vi "数组波形.vi"() -> ()   [LabVIEW 2018]
uses:
  <vilib>/measure/NI_MABase.lvlib
panel:
  out "Dynamic Data Type":dynamicdata(graph) caption="动态数据类型"
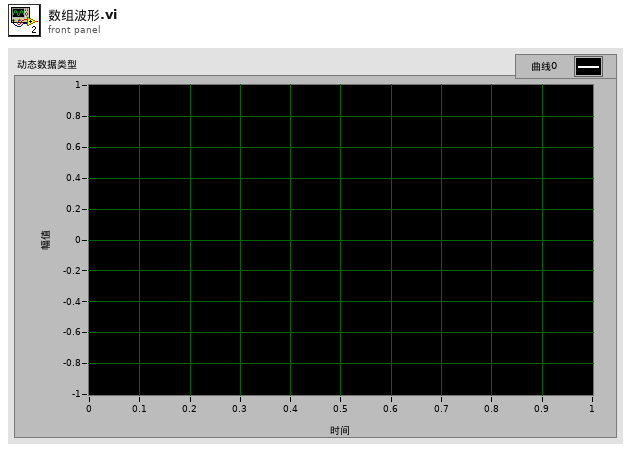
[diagram p1: front panel]
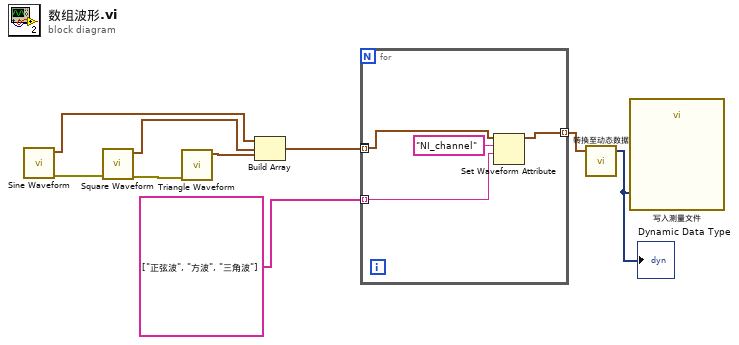
[diagram p0: block diagram]
diagram:
  n1 = call <vilib>:"Sine Waveform.vi"() -> ("error out"=w8:errorcluster, "signal out"=w7:waveform(dbl))  [unwired: 10 in]
  n2 = call <vilib>:"Square Waveform.vi"("error in (no error)"=w8) -> ("error out"=w9:errorcluster, "signal out"=w6:waveform(dbl))  [unwired: 9 in]
  n3 = call <vilib>:"Triangle Waveform.vi"("error in (no error)"=w9) -> ("signal out"=w5:waveform(dbl))  [unwired: 9 in, 1 out]
  n4 = Build Array(w7, w6, w5) -> (w4:waveform(dbl)[])
  n5 = for {
    tunnel: [w10] -> _ mode=indexing
    tunnel: w4 -> [w10] mode=indexing
    tunnel: string[] ["正弦波", "方波", "三角波"] -> [w13] mode=indexing
    tunnel: [w12] -> w2 mode=indexing
    n6 = Set Waveform Attribute(5:w13, 6:"NI_channel" ("名称"), 7:w10) -> (3:w12:waveform(dbl))  [unwired: 1 in, 2 out]
  }
  n7 = call "转换至动态数据"("Array of Waveforms"=w2) -> ("Dynamic Data Type"=w1:dynamicdata)  [unwired: 3 in]
  "Dynamic Data Type" <- w1
  n8 = call "写入测量文件"("Signals"=w1) -> ()  [unwired: 16 in, 3 out]
